vi "AddDocument.vi"(8 "error in":errorcluster, 10 "FilePath":path, 11 "StepRun in":refnum<class "StepRun.lvclass">) -> (0 "error out":errorcluster, 2 "Document":refnum<class "Document.lvclass">, 3 "StepRun out":refnum<class "StepRun.lvclass">)   [LabVIEW 2021, in "ProligentXMLGenerator.lvlib" / "StepRun.lvclass"]
doc: "A document defines a link to an external file. This document is uniquely identified by its Identifier.\nThe document also has an optional Name attribute which is meant to contain a human-friendly identifier, and a FileName attribute. The FileName is used to identify the type of document and should contain an extension so that the appropriate application is launched when the user requests to view the document content.\nAn optional Description can also be specified.\n \nDocuments are unique among siblings by their Identifier property. This makes it possible for two different entities (ex: two different product units) to refer to the same document."
uses:
  StepRun.lvclass
  StepRun.lvclass/StepRun.ctl
  Model/Document/Document.lvclass
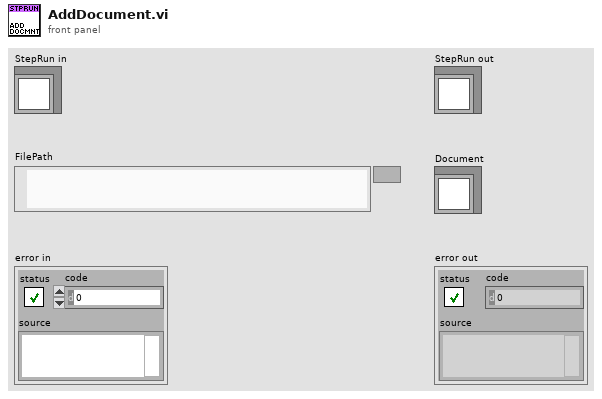
[diagram p1: front panel]
types:
  T1 = typedef "ProligentXMLGenerator.lvlib/StepRun.lvclass/Data.ctl" = cluster{"Name":string, "Measures":refnum<class "Measure.lvclass">[], "FailureReferences":refnum<class "FailureReference.lvclass">[], "Characteristics":refnum<class "Characteristic.lvclass">[], "Documents":refnum<class "Document.lvclass">[], "CustomData":refnum<class "CustomData.lvclass">, "StepExecutionStatus":refnum<class "ExecutionStatus.lvclass">, "StepRunId":refnum<class "Guid.lvclass">, "StepName":refnum<class "NonEmptyString_255.lvclass">, "StartDate":refnum<class "DateTime.lvclass">, "EndDate":refnum<class "DateTime.lvclass">, "TimeZoneInfoId":string}
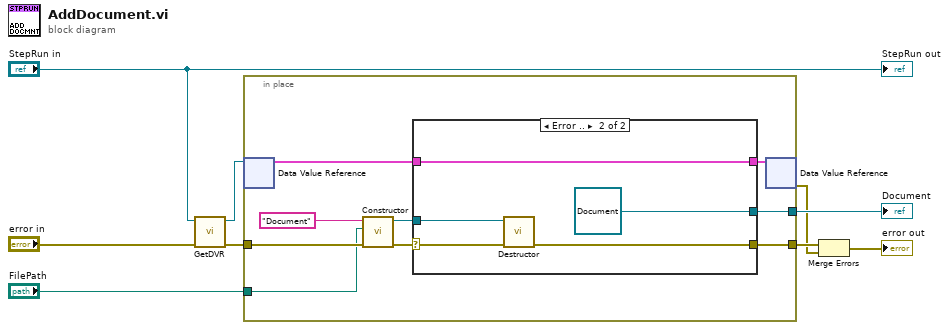
[diagram p0: block diagram]
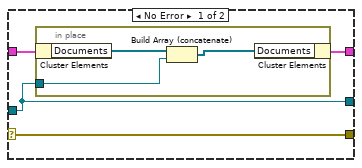
[diagram p2: hidden frame]
diagram:
  n1 = call "GetDVR.vi"("error in"="error in", "StepRun"="StepRun in") -> ("error out"=w4:errorcluster, "DVRReference"=w3:refnum<data-value>)  [unwired: 8 in]
  n2 = in-place "In Place Element Structure" {
    in-place-border: [w18] -> w5
    in-place-border: w4 -> [w11]
    in-place-border: [w15] -> w6
    in-place-border: "FilePath" -> [w10]
    n3 = in-place-dvr #1(w3) -> (w17:T1)  [unwired: 1 out]
    n4 = call "Constructor.vi"("error in (no error)"=w11, "FilePath"=w10, "Name"="Document") -> ("error out"=w13:errorcluster, "DocumentType out"=w14:refnum<class "Document.lvclass">)  [unwired: 7 in]
    n5 = case shown="Error .." w13 {
      selector: w13 -> [w22 w29]
      tunnel: [w19 w30] -> w16
      tunnel: [w22 w28] -> w18
      tunnel: w14 -> [w21 w27]
      tunnel: w17 -> [w20 w30]
      tunnel: [w21 refnum<class "Document.lvclass"> refnum ("ProligentResultProcessor:DocumentType")] -> w15
      frame No Error {
        n6 = in-place "In Place Element Structure" {
          in-place-border: w21 -> [w25]
          n7 = in-place-cluster #2(w20) -> ("Documents"=w24:refnum<class "Document.lvclass">[])
          n8 = Build Array (concatenate)(w24, w25) -> (w23:refnum<class "Document.lvclass">[])
          n9 = in-place-cluster #2("Documents"=w23) -> (w19:T1)
        }
      }
      frame Error {
        n10 = call "Destructor.vi"("error in"=w29, "Document in"=w27) -> ("error out"=w28:errorcluster)  [unwired: 9 in]
      }
    }
    n11 = in-place-dvr #1(w16) -> (w2:errorcluster)  [unwired: 1 out]
  }
  "Document" <- w6
  n12 = Merge Errors(w5, w2) -> (→"error out":errorcluster)
  "StepRun out" <- "StepRun in"
